vi "Read Waveform Increment.vi"(11 "AO in":refnum<class "Analog Output.lvclass">) -> (3 "increment":u32)   [LabVIEW 2017, in "Analog IO.lvlib" / "Analog Output.lvclass"]
uses:
  Analog Output.lvclass
  Analog Output.lvclass/Analog Output.ctl
  <vilib>/rvi/DataTransferAndStorage/Container/Common/niFpgaContainerExecOnDevCompGetState.vi
  <vilib>/rvi/Emulation/niFpgaEmulationIsFPGAContextNoSignature.vi
  <vilib>/rvi/DataTransferAndStorage/Container/Common/niFpgaContainerGetUniqueNameForEmu.vi
  <vilib>/rvi/eio/common/nirviEmuReportErrorAndStop.vi
  <vilib>/rvi/Emulation/niFpgaSctlEmulationGetInTimedLoop.vi
  <vilib>/rvi/Emulation/niFpgaProcessEmulError.vi
  <vilib>/rvi/DataTransferAndStorage/Container/XNode/niFpgaContainer.xnode
  <vilib>/rvi/DataTransferAndStorage/Handshake/Emulation/niFpgaHandshakeEmulationRefIn.vi
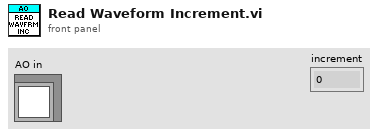
[diagram p1: front panel]
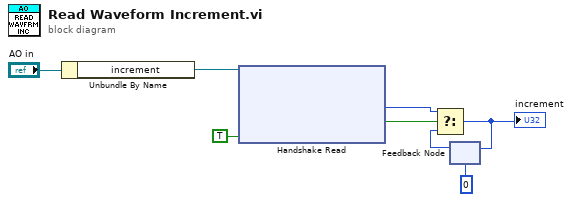
[diagram p0: block diagram]
diagram:
  n1 = Unbundle By Name("AO in") -> ("increment"=w7:refnum<k21>)
  n2 = xnode ("Handshake Read")("Ready for Output"=TRUE, "Handshake In"=w7) -> ("Data"=w5:u32, "Output Valid"=w6:bool)  [unwired: 1 out]
  n3 = feedback #1(u32 0 ("Data")) -> (w4:u32)
  n4 = Select(t=w5, s=w6, f=w4) -> (s? t:f=w3:u32)
  "increment" <- w3
  n5 = feedback-in #1(w3) -> ()
